vi "ContBuildProgamQueue.vi"(9 "Refresh ratio per reactor":dbl=0.08, 10 "Continuous Program":string[][](array[string])) -> (1 "Continuous Program modified":string[][](array[string]))   [LabVIEW 2018, in "ContinousLoop.lvlib"]
uses:
  ContinousLoop.lvlib
panel:
  out "# elements in queue":i32
  out "created new?":bool
  out "elements":T1(array[cluster])
  out "error out":errorcluster
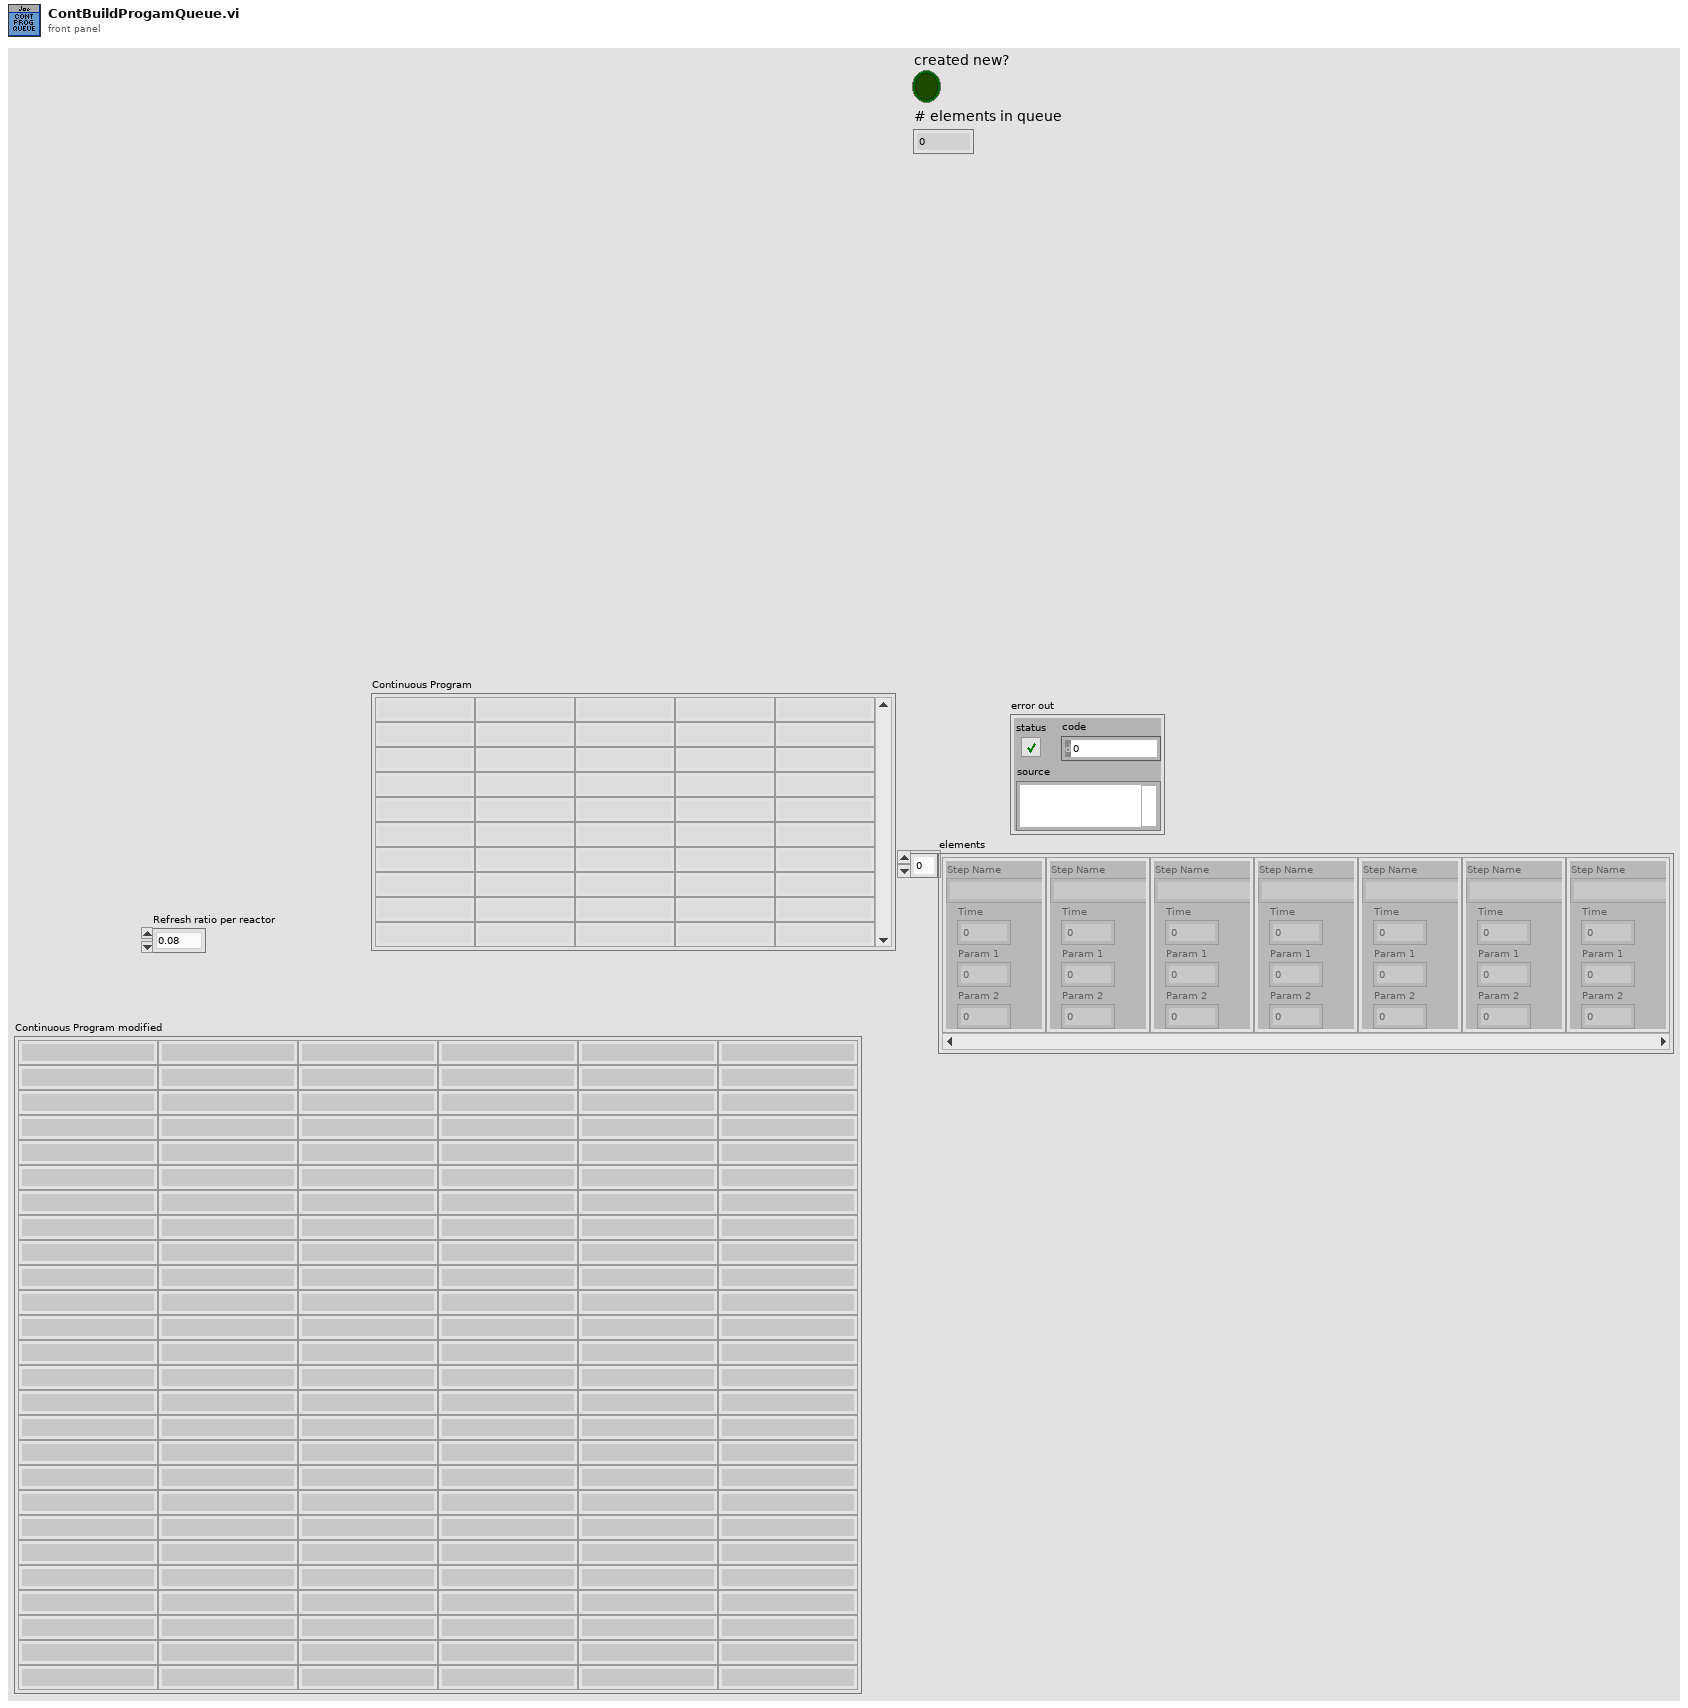
[diagram p1: front panel]
types:
  T1 = cluster{"Step Name":string, "Time":dbl, "Param 1":dbl, "Param 2":i32}[]
  T2 = cluster{"Step Name":string, "Time":dbl, "Param 1":dbl, "Param 2":i32}
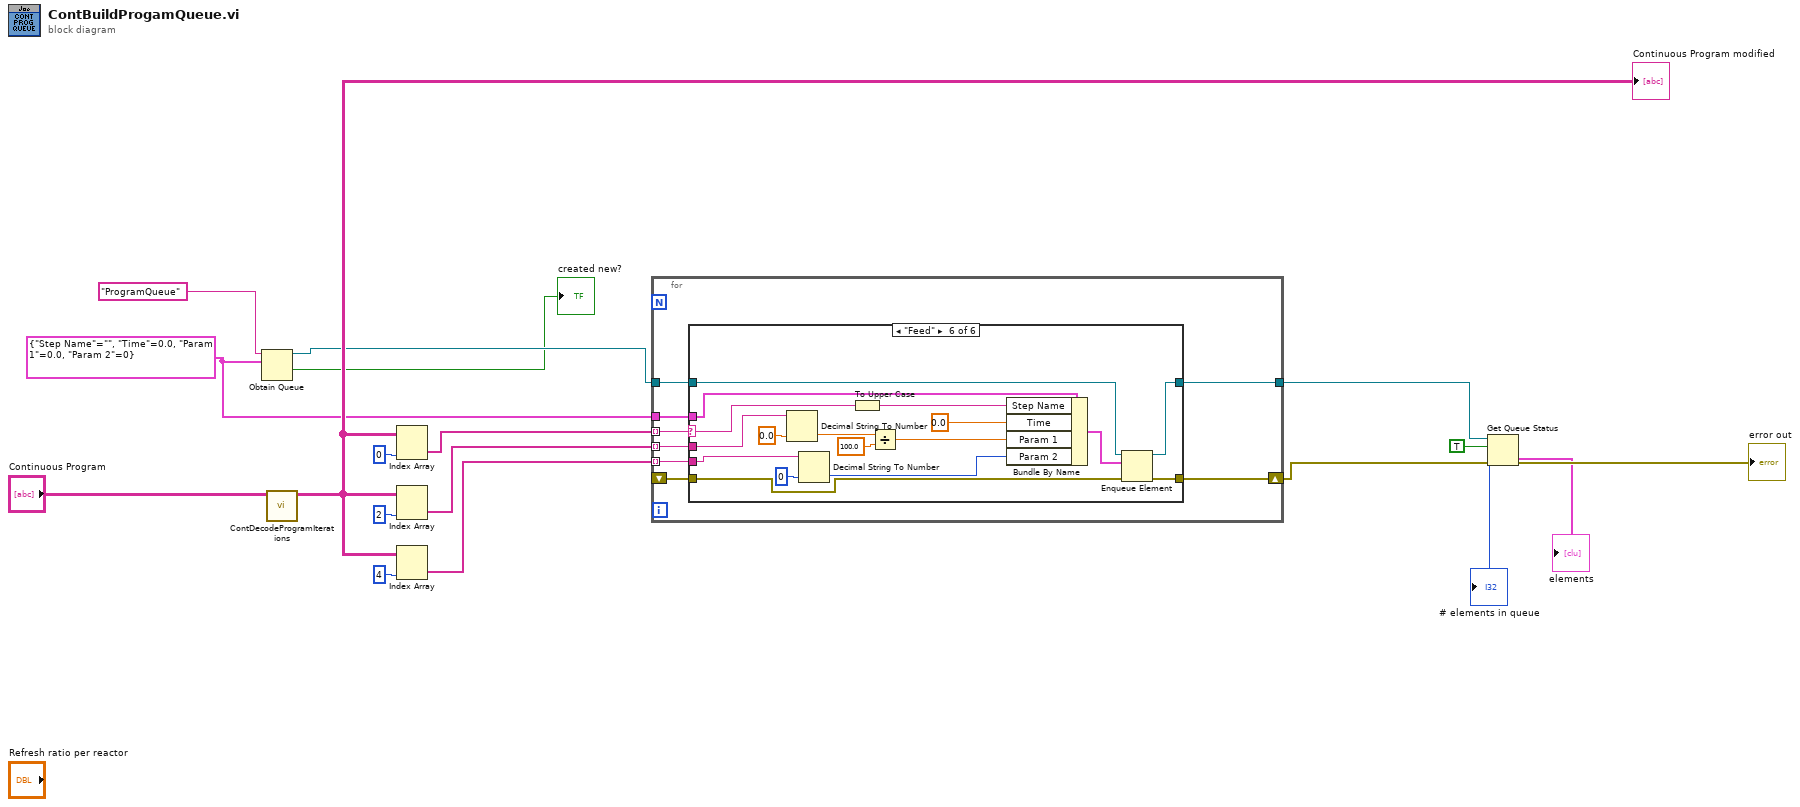
[diagram p0: block diagram]
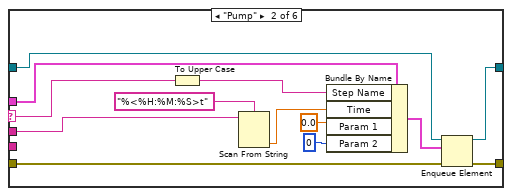
[diagram p3: hidden frame]
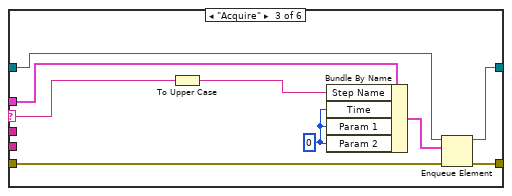
[diagram p4: hidden frame]
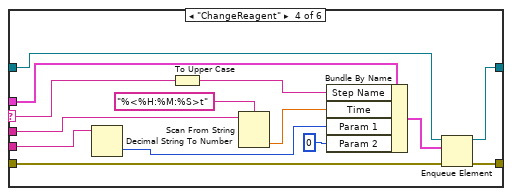
[diagram p5: hidden frame]
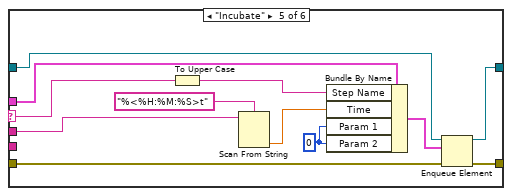
[diagram p6: hidden frame]
diagram:
  w4 = T2 {"Step Name"="", "Time"=0.0, "Param 1"=0.0, "Param 2"=0}
  n1 = Obtain Queue(name (unnamed)="ProgramQueue", element data type=w4) -> (queue out=w5:refnum<queue>, created new?=→"created new?":bool)  [unwired: 3 in, 1 out]
  n2 = call "ContDecodeProgramIterations.vi"("Continuous Program in"="Continuous Program") -> ("Continuous Program out"=w11:string[][])  [unwired: 10 in]
  "Continuous Program modified" <- w11
  n3 = Index Array(array=w11, index (col)=0 ("disabled index (col)")) -> (element=w18:string[])  [unwired: 1 in]
  n4 = Index Array(array=w11, index (col)=2 ("disabled index (col)")) -> (element=w15:string[])  [unwired: 1 in]
  n5 = Index Array(array=w11, index (col)=4 ("disabled index (col)")) -> (element=w13:string[])  [unwired: 1 in]
  n6 = for {
    tunnel: w18 -> [w24] mode=indexing
    tunnel: w15 -> [w26] mode=indexing
    tunnel: w13 -> [w25] mode=indexing
    tunnel: w4 -> [w23]
    shift-right: [w21] -> w8
    shift-left: _ -> [w20]
    tunnel: w5 -> [w22]
    tunnel: [w19] -> w2
    n7 = case shown="\"Feed\"" w24 {
      selector: w24 -> [_ w38 w49 w58 w72 w87]
      tunnel: w26 -> [_ w41 _ w63 w76 w93]
      tunnel: w25 -> [_ _ _ w64 _ w79]
      tunnel: w23 -> [_ w39 w50 w61 w74 w91]
      tunnel: [w28 w31 w43 w55 w71 w90] -> w19
      tunnel: w22 -> [w28 w35 w47 w54 w70 w89]
      tunnel: [w27 w33 w45 w51 w67 w86] -> w21
      tunnel: w20 -> [w27 w32 w44 w52 w68 w78]
      frame Default {
      }
      frame "Pump" {
        n8 = To Upper Case(1:w38) -> (0:w34:string)
        n9 = Scan From String(format string="%<%H:%M:%S>t", input string=w41) -> (output 1=w30:dbl)  [unwired: 3 in, 3 out]
        n10 = Bundle By Name(cluster=w39, "Step Name"=w34, "Time"=w30, "Param 1"=0.0, "Param 2"=0) -> (w37:T2)
        n11 = Enqueue Element(queue=w35, element=w37, error in (no error)=w32) -> (queue out=w31:refnum<queue>, error out=w33:errorcluster)  [unwired: 1 in, 1 out]
      }
      frame "Acquire" {
        w42 = 0
        n12 = To Upper Case(1:w49) -> (0:w46:string)
        n13 = Bundle By Name(cluster=w50, "Step Name"=w46, "Time"=w42, "Param 1"=w42, "Param 2"=w42) -> (w48:T2)
        n14 = Enqueue Element(queue=w47, element=w48, error in (no error)=w44) -> (queue out=w43:refnum<queue>, error out=w45:errorcluster)  [unwired: 1 in, 1 out]
      }
      frame "ChangeReagent" {
        n15 = Decimal String To Number(string=w64) -> (number=w60:i32)  [unwired: 2 in, 1 out]
        n16 = To Upper Case(1:w58) -> (0:w53:string)
        n17 = Scan From String(format string="%<%H:%M:%S>t", input string=w63) -> (output 1=w59:dbl)  [unwired: 3 in, 3 out]
        n18 = Bundle By Name(cluster=w61, "Step Name"=w53, "Time"=w59, "Param 1"=w60, "Param 2"=0) -> (w57:T2)
        n19 = Enqueue Element(queue=w54, element=w57, error in (no error)=w52) -> (queue out=w55:refnum<queue>, error out=w51:errorcluster)  [unwired: 1 in, 1 out]
      }
      frame "Incubate" {
        w66 = 0
        n20 = To Upper Case(1:w72) -> (0:w69:string)
        n21 = Scan From String(format string="%<%H:%M:%S>t", input string=w76) -> (output 1=w73:dbl)  [unwired: 3 in, 3 out]
        n22 = Bundle By Name(cluster=w74, "Step Name"=w69, "Time"=w73, "Param 1"=w66, "Param 2"=w66) -> (w65:T2)
        n23 = Enqueue Element(queue=w70, element=w65, error in (no error)=w68) -> (queue out=w71:refnum<queue>, error out=w67:errorcluster)  [unwired: 1 in, 1 out]
      }
      frame "Feed" {
        n24 = Decimal String To Number(string=w93, default (0L)=0.0 ("default (0 I32)")) -> (number=w82:dbl)  [unwired: 1 in, 1 out]
        n25 = Decimal String To Number(string=w79, default (0L)=i16 0 ("default (0 I32)")) -> (number=w77:i16)  [unwired: 1 in, 1 out]
        n26 = To Upper Case(1:w87) -> (0:w88:string)
        n27 = Divide(x=w82, y=100.0) -> (x/y=w83:dbl)
        n28 = Bundle By Name(cluster=w91, "Step Name"=w88, "Time"=0.0, "Param 1"=w83, "Param 2"=w77) -> (w92:T2)
        n29 = Enqueue Element(queue=w89, element=w92, error in (no error)=w78) -> (queue out=w90:refnum<queue>, error out=w86:errorcluster)  [unwired: 1 in, 1 out]
      }
    }
  }
  n30 = Get Queue Status(queue=w2, return elements? (F)=TRUE, error in (no error)=w8) -> (error out=→"error out":errorcluster, # elements in queue=→"# elements in queue":i32, elements=→"elements":T1)  [unwired: 5 out]
